vi "SetRTLED.vi"(8 "error in (no error)":errorcluster, 11 "LED state":bool) -> (0 "error out":errorcluster, 3 "LED state":bool)   [LabVIEW 2017, in "BlinkProcess.lvlib"]
uses:
  <vilib>/addons/BlinkProcess/BlinkProcess.lvlib
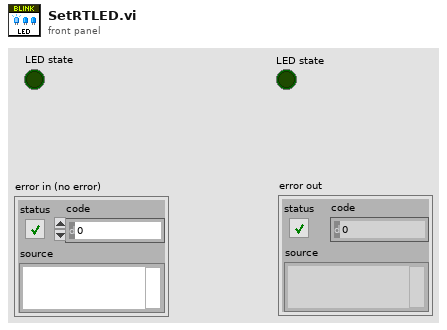
[diagram p1: front panel]
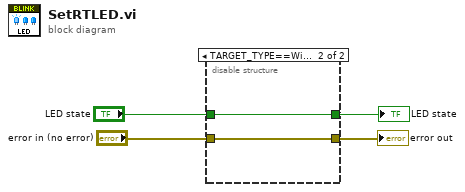
[diagram p0: block diagram]
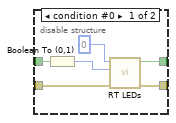
[diagram p2: hidden frame]
diagram:
  n1 = disable-structure shown="TARGET_TYPE==Windows" {
    disable-tunnel: "error in (no error)" -> [w8 w11]
    disable-tunnel: "LED state" -> [w7 w12]
    disable-tunnel: [w6 w11] -> w2
    disable-tunnel: [w5 w12] -> w1
    frame condition #0 {
      n2 = Boolean To (0,1)(Boolean=w7) -> (0, 1=w10:i16)
      n3 = call <vilib>:"RT LEDs.vi"("error in (no error)"=w8, "State"=w10, "LED Num"=0) -> ("error out"=w6:errorcluster, "Led State"=w5:bool)  [unwired: 3 in]
    }
    frame condition #1 (active) {
    }
  }
  "error out" <- w2
  "LED state" <- w1
